vi "Fade_Into_Color.vi"(8 "Length":dbl, 9 "Color_Goal":u32(colorbox)=16776002, 10 "Color_Start":u32(colorbox)=16776002, 11 "fade constant":dbl) -> (3 "Output_Array":u32[](array[colorbox]))   [LabVIEW 2020]
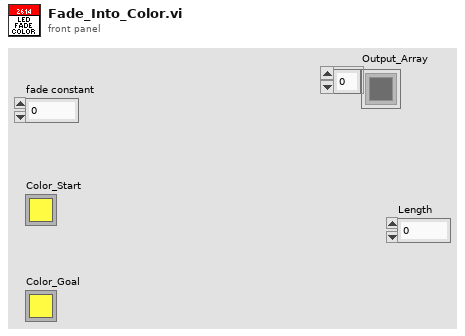
[diagram p1: front panel]
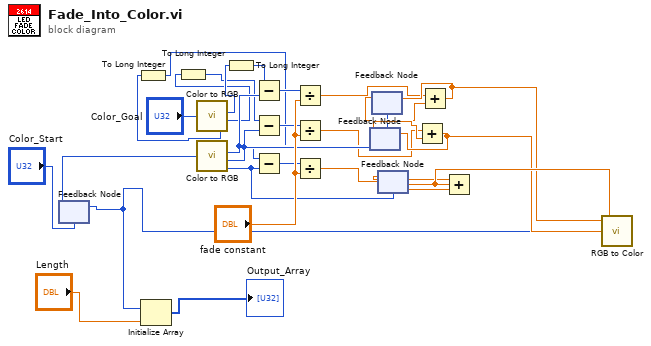
[diagram p0: block diagram]
diagram:
  n1 = feedback #1("Color_Start") -> (w6:u32)
  n2 = call <vilib>:"Color to RGB.vi"("Color"="Color_Goal") -> ("R"=w14:u8, "G"=w12:u8, "B"=w10:u8)  [unwired: 1 out]
  n3 = To Long Integer(number=w10) -> (32bit integer=w9:i32)
  n4 = To Long Integer(number=w12) -> (32bit integer=w11:i32)
  n5 = call <vilib>:"Color to RGB.vi"("Color"=w6) -> ("R"=w19:u8, "G"=w22:u8, "B"=w25:u8)  [unwired: 1 out]
  n6 = To Long Integer(number=w14) -> (32bit integer=w13:i32)
  n7 = Subtract(x=w13, y=w19) -> (x-y=w16:i32)
  n8 = Subtract(x=w11, y=w22) -> (x-y=w17:i32)
  n9 = Subtract(x=w9, y=w25) -> (x-y=w18:i32)
  n10 = Divide(x=w16, y="fade constant") -> (x/y=w5:dbl)
  n11 = Divide(x=w17, y="fade constant") -> (x/y=w4:dbl)
  n12 = Divide(x=w18, y="fade constant") -> (x/y=w3:dbl)
  n13 = feedback #2(w22) -> (w23:dbl)
  n14 = feedback #3(w19) -> (w20:dbl)
  n15 = feedback #4(w25) -> (w26:dbl)
  n16 = Add(x=w4, y=w23) -> (x+y=w24:dbl)
  n17 = feedback-in #2(w24) -> ()
  n18 = Add(x=w5, y=w20) -> (x+y=w21:dbl)
  n19 = feedback-in #3(w21) -> ()
  n20 = Add(x=w26, y=w3) -> (x+y=w27:dbl)
  n21 = feedback-in #4(w27) -> ()
  n22 = call <vilib>:"RGB to Color.vi"("B"=w27, "G"=w24, "R"=w21) -> ("Color"=w7:u32)
  n23 = feedback-in #1(w7) -> ()
  n24 = Initialize Array(w7, "Length") -> (→"Output_Array":u32[])
